vi "Test_InsertVI.vi"(11 "Event Registration Refnum":refnum<event-registration>) -> ()   [LabVIEW 2021]
panel:
  out "Waveform Chart":dbl(graph)
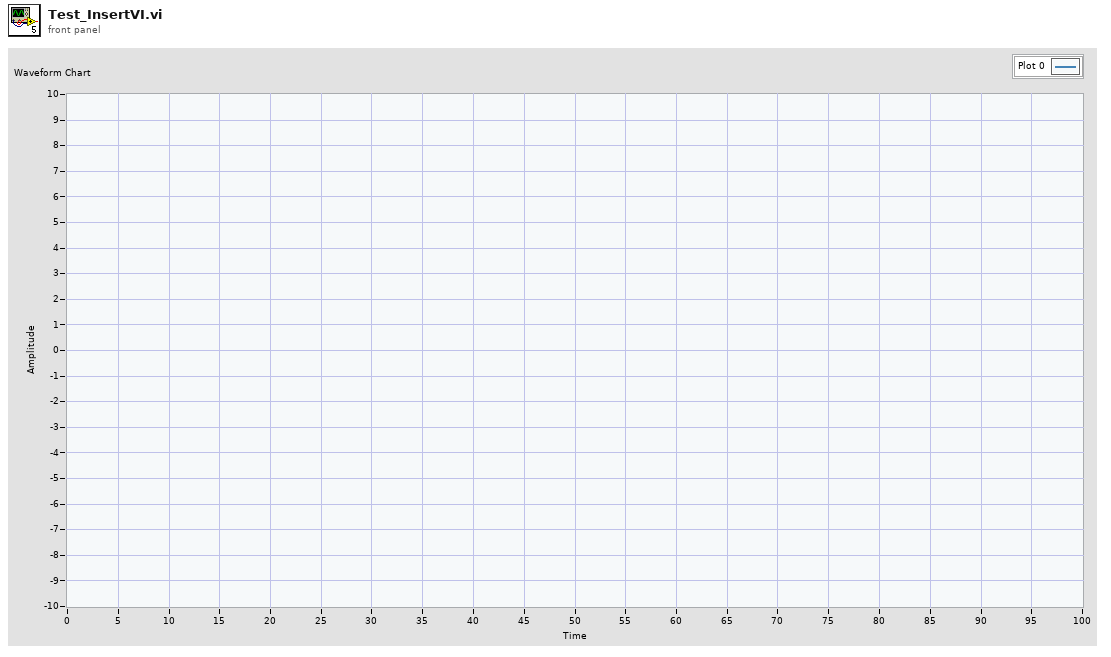
[diagram p1: front panel]
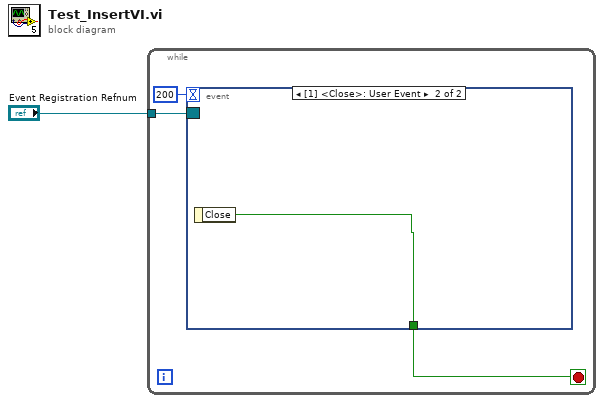
[diagram p0: block diagram]
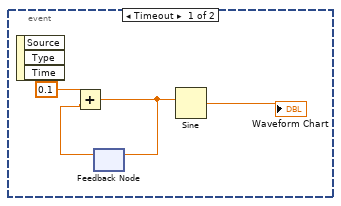
[diagram p2: hidden frame]
diagram:
  n1 = while {
    tunnel: "Event Registration Refnum" -> [w3]
    stop <- w2 stop-if-true
    n2 = event shown="[1] <Close>: User Event" {
      selector: w3 -> [_ _]
      dyn-events: _ -> [_ _]
      timeout: 200 -> [_ _]
      tunnel: [_ w9] -> w2
      event Timeout {
        n3 = event-data() -> ()  [unwired: 1 in, 3 out]
        n4 = feedback #1() -> (w5:dbl)  [unwired: 1 in]
        n5 = Add(x=0.1, y=w5) -> (x+y=w6:dbl)
        n6 = feedback-in #1(w6) -> ()
        n7 = Sine(x=w6) -> (sin(x)=→"Waveform Chart":dbl)
      }
      event User Event {
        n8 = event-data() -> ("Close"=w9:bool)  [unwired: 1 in]
      }
    }
  }
